vi "Get SMO Database Paths.vi"(5 "getAll Cluster":variant, 7 "Default Paths":string, 8 "error in (no error)":errorcluster, 11 "instrument.PPMS in":refnum<class "instrument.PPMS-W-1.lvclass">) -> (0 "error out":errorcluster, 2 "Paths":string, 3 "instrument.PPMS out":refnum<class "instrument.PPMS-W-1.lvclass">)   [LabVIEW 2019, in "instrument.PPMS-W-1.lvclass"]
uses:
  instrument.PPMS-W-1.lvclass
  instrument.PPMS/Typedefs/PPMS.getAll--cluster.ctl
  instrument.PPMS/instrument.PPMS.lvclass
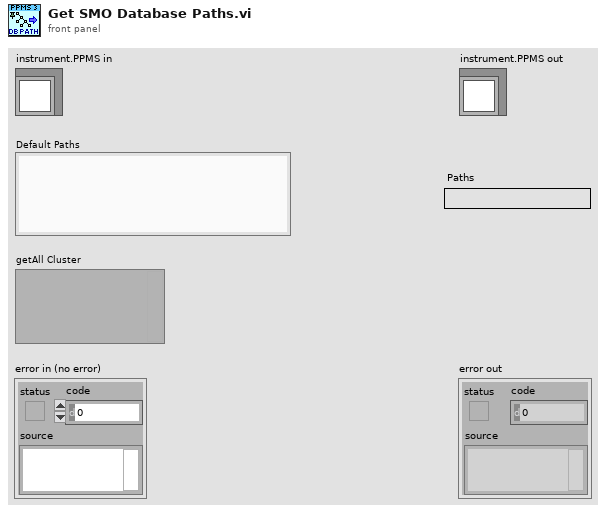
[diagram p1: front panel]
types:
  T1 = typedef "instrument.PPMS.lvclass/PPMS.getAll--cluster.ctl" = cluster{"Chamber Status":string, "Helium Level":dbl, "Temperature":dbl, "Temperature Status":string, "Magnetic Field":dbl, "Magnet Status":string, "Position":dbl}
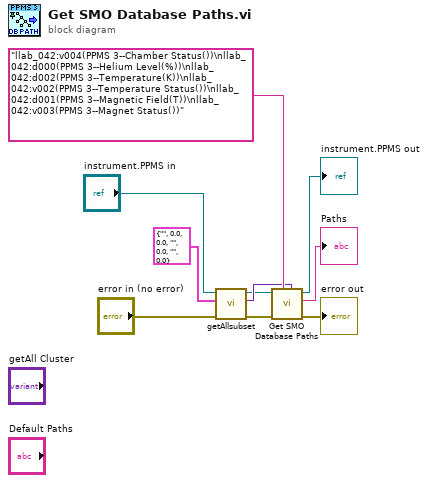
[diagram p0: block diagram]
diagram:
  n1 = call-dynamic "getAllsubset.vi"("error in (no error)"="error in (no error)", "getAll"=T1 {"Chamber Status"="", "Helium Level"=0.0, "Temperature"=0.0, "Temperature Status"="", "Magnetic Field"=0.0, "Magnet Status"="", "Position"=0.0}, "instrument.PPMS3 in"="instrument.PPMS in") -> ("error out"=w2:errorcluster, "output cluster"=w5:variant, "instrument.PPMS3 out"=w1:refnum<class "instrument.PPMS-W-1.lvclass">)  [unwired: 6 in]
  n2 = call-parent "Get SMO Database Paths.vi"("getAll Cluster"=w5, "Default Paths"="llab_042:v004(PPMS 3--Chamber Status())\nllab_042:d000(PPMS 3--Helium Level(%))\nllab_042:d002(PPMS 3--Temperature(K))\nllab_042:v002(PPMS 3--Temperature Status())\nllab_042:d001(PPMS 3--Magnetic Field(T))\nllab_042:v003(PPMS 3--Magnet Status())" ("Paths"), "error in (no error)"=w2, "instrument.PPMS in"=w1) -> ("error out"=→"error out":errorcluster, "Paths"=→"Paths":string, "instrument.PPMS out"=→"instrument.PPMS out":refnum<class "instrument.PPMS-W-1.lvclass">)  [unwired: 5 in]
